vi "Get Status.vi"(8 "error in (no error)":errorcluster, 11 "Filter Wheel in":refnum<class "Filter Wheel.lvclass">) -> (0 "error out":errorcluster, 2 "FW Status":T1={"State"=enum."Move Complete", "Positions"=[], "Names"=[], "Notch"=[], "Moving"=[FALSE, FALSE]}, 3 "Filter Wheel out":refnum<class "Filter Wheel.lvclass">)   [LabVIEW 2021, in "Filter Wheel.lvclass"]
uses:
  Filter Wheel.lvclass
  FW cluster Status.ctl
  FW enum status.ctl
  Filter Wheel.lvclass/Filter Wheel.ctl
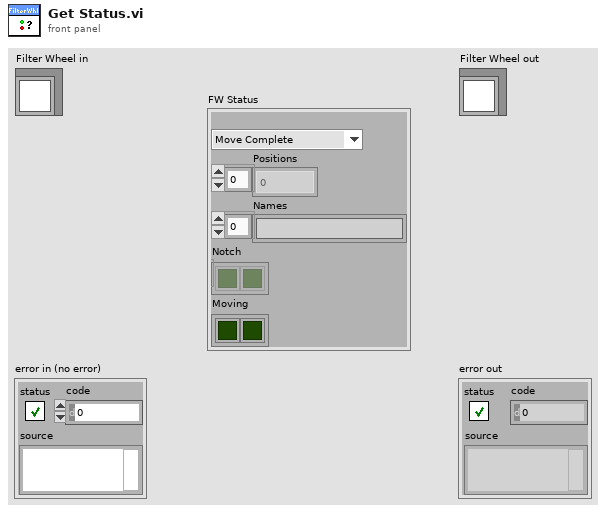
[diagram p1: front panel]
types:
  T1 = typedef "FW cluster Status.ctl" = cluster{"State":T2, "Positions":i32[], "Names":string[], "Notch":bool[], "Moving":bool[]}
  T2 = typedef "FW enum status.ctl" = enum16{"Initializing", "Moving", "Move Complete", "Error"}
  T3 = typedef "Filter Wheel.lvclass/Filter Wheel Details.ctl" = cluster{"Names":string[], "Relative Position":i32[], "Wheel Name":string}
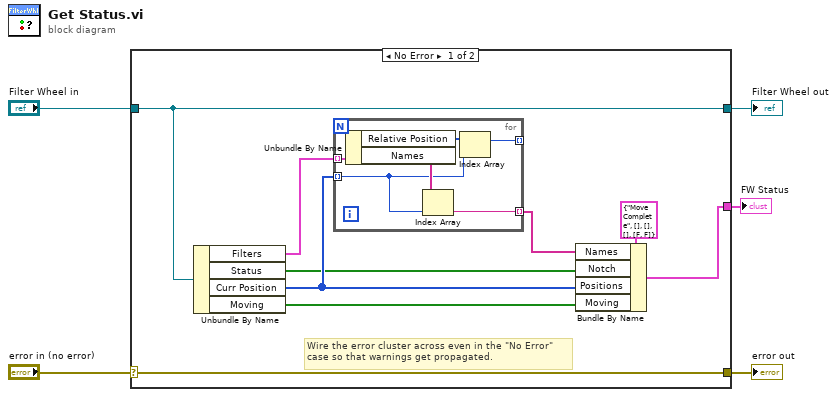
[diagram p0: block diagram]
diagram:
  n1 = case shown="No Error" "error in (no error)" {
    selector: "error in (no error)" -> [w14 w22]
    tunnel: [w14 w22] -> w4
    tunnel: [w10 w21] -> w2
    tunnel: "Filter Wheel in" -> [w10 w21]
    tunnel: [w11 _] -> w1
    frame No Error {
      # "Wire the error cluster across even in the \"No Error\"\ncase so that warnings get propagated."
      n2 = Unbundle By Name(w10) -> ("Filters"=w12:T3[], "Status"=w7:bool[], "Curr Position"=w8:i32[], "Moving"=w6:bool[])
      n3 = for {
        tunnel: w12 -> [w20] mode=indexing
        tunnel: w8 -> [w15] mode=indexing
        tunnel: [w18] -> w9 mode=indexing
        tunnel: [w16] -> _ mode=indexing
        n4 = Unbundle By Name(w20) -> ("Relative Position"=w17:i32[], "Names"=w19:string[])
        n5 = Index Array(array=w19, index=w15) -> (element=w18:string)
        n6 = Index Array(array=w17, index=w15) -> (element=w16:i32)
      }
      n7 = Bundle By Name(cluster=T1 {"State"=enum."Move Complete", "Positions"=[], "Names"=[], "Notch"=[], "Moving"=[FALSE, FALSE]}, "Names"=w9, "Notch"=w7, "Positions"=w8, "Moving"=w6) -> (w11:T1)
    }
    frame Error {
    }
  }
  "error out" <- w4
  "Filter Wheel out" <- w2
  "FW Status" <- w1
